vi "all variables to string.vi"() -> ()   [LabVIEW 2012]
panel:
  out "Variable Name":string
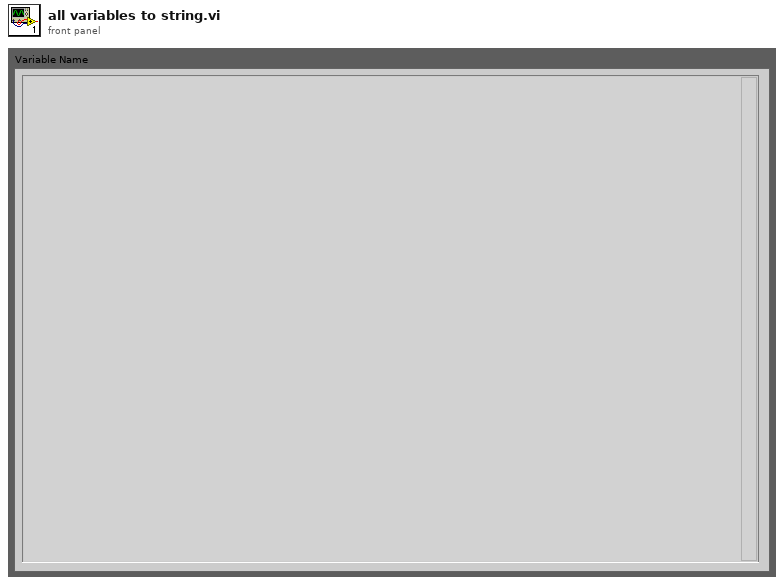
[diagram p1: front panel]
types:
  T1 = typedef "VariantType.lvlib/Type.ctl" = enum8{"Invalid Type", "Void", "I8", "I16", "I32", "I64", "U8", "U16", "U32", "U64", "Single Float", "Double Float", "Extended Float", "Single Complex", "Double Complex", "Extended Complex", "Enum U8", "Enum U16", "Enum U32", "Enum U64", "Single Float With Unit", "Double Float With Unit", "Extended Float With Unit", "Single Complex with Unit", "Double Complex with Unit", "Extended Complex with Unit", "Boolean", "String", "Path", "Picture", "Tag", "Array", "Cluster", "Variant", "LV Variant", "Waveform", "Timestamp", "Digital Waveform", "Digital Data", "ExpressData", "Refnum", "External Data", "VI", "Poly VI", "LabVIEW Class Instance", "Fixed Point"}
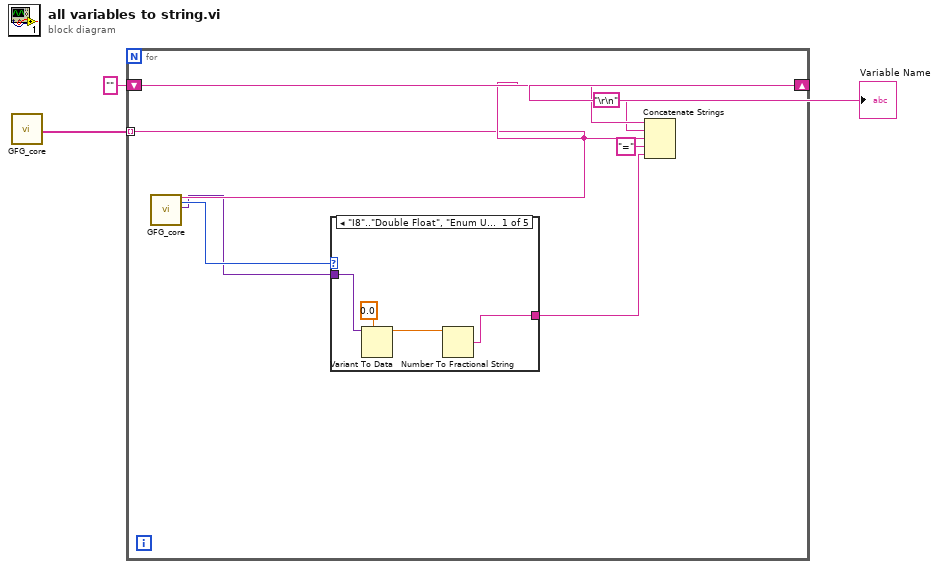
[diagram p0: block diagram]
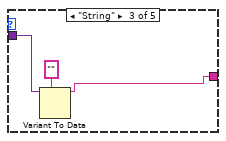
[diagram p3: hidden frame]
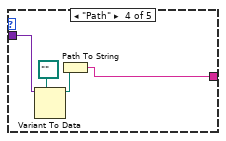
[diagram p4: hidden frame]
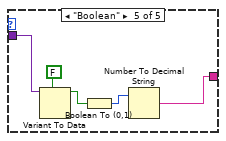
[diagram p5: hidden frame]
diagram:
  n1 = call "GFG_core.vi"() -> ("All Variable Names Out"=w3:string[])  [unwired: 13 in, 6 out]
  n2 = for {
    tunnel: w3 -> [w8] mode=indexing
    shift-right: [w9] -> w1
    shift-left: "" -> [w11]
    n3 = call "GFG_core.vi"("Variable Name in"=w8) -> ("Data Type Out"=w6:T1, "Variant Out"=w5:variant)  [unwired: 12 in, 5 out]
    n4 = case shown="\"I8\"..\"Double Float\", \"Enum U8\"..\"Enum U64\"" w6 {
      tunnel: w5 -> [w14 _ w18 w22 w27]
      tunnel: [w12 _ w16 w19 w23] -> w4
      frame "I8".."Double Float", "Enum U8".."Enum U64" {
        n5 = Variant To Data(type=0.0, Variant=w14) -> (data=w13:dbl)  [unwired: 1 in, 1 out]
        n6 = Number To Fractional String(number=w13) -> (F-format string=w12:string)  [unwired: 3 in]
      }
      frame Default {
      }
      frame "String" {
        n7 = Variant To Data(type="" ("Variable Name Out"), Variant=w18) -> (data=w16:string)  [unwired: 1 in, 1 out]
      }
      frame "Path" {
        n8 = Variant To Data(type=path "" ("configuration file path 2"), Variant=w22) -> (data=w20:path)  [unwired: 1 in, 1 out]
        n9 = Path To String(path=w20) -> (string=w19:string)
      }
      frame "Boolean" {
        n10 = Variant To Data(type=FALSE, Variant=w27) -> (data=w25:bool)  [unwired: 1 in, 1 out]
        n11 = Boolean To (0,1)(Boolean=w25) -> (0, 1=w24:i16)
        n12 = Number To Decimal String(number=w24) -> (decimal integer string=w23:string)  [unwired: 1 in]
      }
    }
    n13 = Concatenate Strings(w11, "\r\n", w8, "=" ("string"), w4) -> (w9:string)
  }
  "Variable Name" <- w1
